vi "Configure Trigger AND Qualifier.vi"(0 "VISA resource name":refnum<visa-resource-name>, 1 "Enable AND Qualifier (F: Disable)":bool, 5 "Channel (1: Channel1)":i32(ring)=1 items=["Channel1"=1, "Channel2"=2, "Channel3"=3, "Channel4"=4], 9 "Logical Value (0: High)":i32(ring) items=["High", "Low", "Don't Care"], 11 "error in (no error)":errorcluster) -> (4 "VISA resource name out":refnum<visa-resource-name>, 15 "error out":errorcluster)   [LabVIEW 2020, in "Agilent 90000 Series.lvlib"]
doc: "Configure trigger AND qualifier."
uses:
  Agilent 90000 Series.lvlib
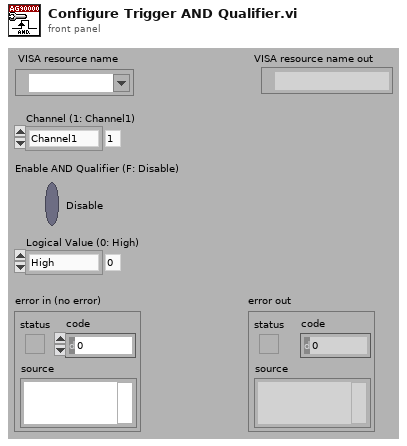
[diagram p1: front panel]
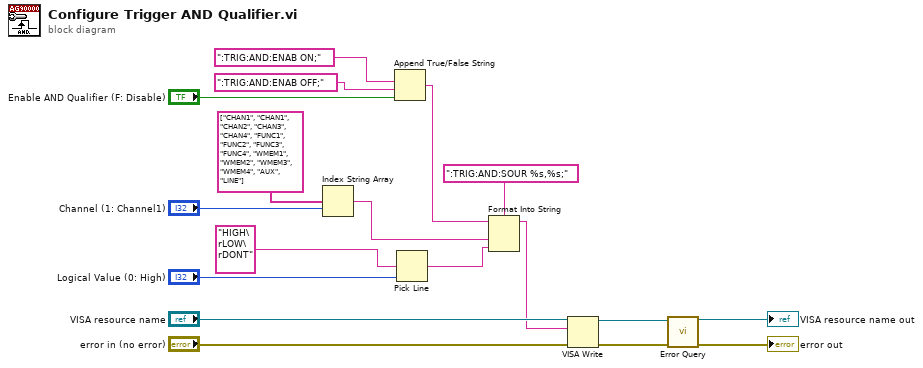
[diagram p0: block diagram]
diagram:
  n1 = Index String Array(1:"Channel (1: Channel1)", 2:string[] ["CHAN1", "CHAN1", "CHAN2", "CHAN3", "CHAN4", "FUNC1", "FUNC2", "FUNC3", "FUNC4", "WMEM1", "WMEM2", "WMEM3", "WMEM4", "AUX", "LINE"]) -> (0:w3:string)  [unwired: 1 out]
  n2 = Append True/False String(1:"Enable AND Qualifier (F: Disable)", 2:":TRIG:AND:ENAB OFF;", 3:":TRIG:AND:ENAB ON;") -> (0:w2:string)  [unwired: 1 out]
  n3 = Pick Line(multi-line string="HIGH\rLOW\rDONT", line index="Logical Value (0: High)") -> (output string=w15:string)  [unwired: 1 out]
  n4 = Format Into String(format string=":TRIG:AND:SOUR %s,%s;", initial string=w2, w3, w15) -> (resulting string=w1:string)  [unwired: 1 in, 1 out]
  n5 = VISA Write(VISA resource name="VISA resource name", write buffer=w1, error in (no error)="error in (no error)") -> (VISA resource name out=w9:refnum<visa-resource-name>, error out=w8:errorcluster)  [unwired: 1 out]
  n6 = call "Error Query.vi"("error in (no error)"=w8, "VISA resource name"=w9) -> ("error out"=→"error out":errorcluster, "VISA resource name out"=→"VISA resource name out":refnum<visa-resource-name>)  [unwired: 8 out]
